vi "simx Read Vision Sensor.vi"(0 "clientID":i32, 1 "auxValuesCount":i32, 5 "sensorHandle":i32, 7 "detectionState":string, 9 "auxValues":sgl, 11 "error in (no error)":errorcluster, 12 "operationMode":i32) -> (3 "auxValuesCount out":i32, 4 "function return":i32, 8 "detectionState out":string, 10 "auxValues out":sgl, 15 "error out":errorcluster)   [LabVIEW 2019, in "PXL_V-REP.lvlib"]
doc: "EXTAPI_DLLEXPORT simxInt simxReadVisionSensor(simxInt clientID,simxInt sensorHandle,simxUChar* detectionState,simxFloat** auxValues,simxInt** auxValuesCount,simxInt operationMode);"
uses:
  PXL_V-REP.lvlib
  <userlib>/V-REP/remoteApi.dll
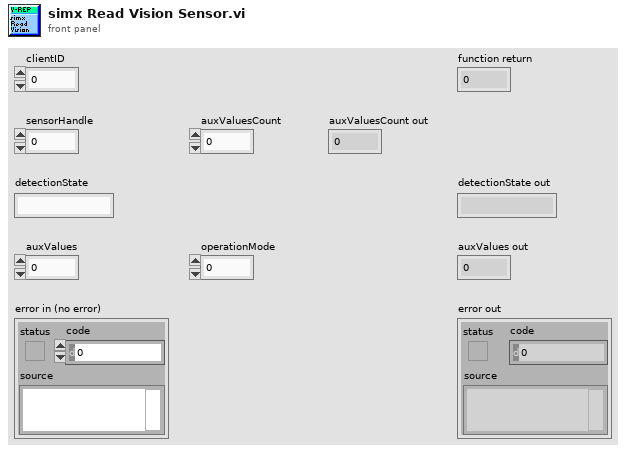
[diagram p1: front panel]
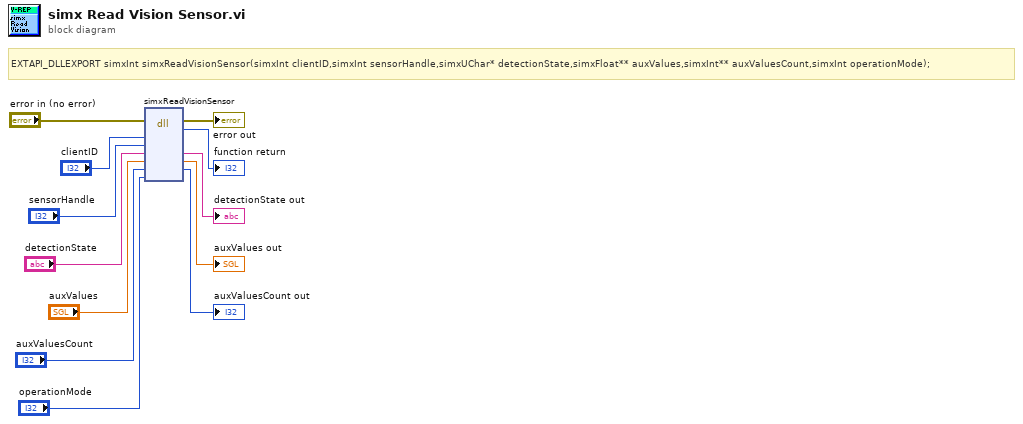
[diagram p0: block diagram]
diagram:
  # "EXTAPI_DLLEXPORT simxInt simxReadVisionSensor(simxInt clientID,simxInt sensorHandle,simxUChar* detectionState,simxFloat** auxValues,simxInt** auxValuesCount,simxInt operationMode);"
  n1 = dll-call lib="C:/Program Files (x86)/National Instruments/LabVIEW 2019/user.lib/V-REP/remoteApi.*" fn="simxReadVisionSensor"(error in="error in (no error)", "clientID"="clientID", "sensorHandle"="sensorHandle", "detectionState"="detectionState", "auxValues"="auxValues", "auxValuesCount"="auxValuesCount", "operationMode"="operationMode") -> (error out=→"error out":errorcluster, →"function return":i32, "detectionState"=→"detectionState out":string, "auxValues"=→"auxValues out":sgl, "auxValuesCount"=→"auxValuesCount out":i32)  [unwired: 5 in, 1 out]
